vi "Ans_Step2.vi"   [LabVIEW 2012]
uses:
  <vilib>/NXT/Subs/MotorOutput.ctl
types:
  T1 = typedef "MotorOutput.ctl" = u8
  T2 = typedef "LVHSConnector.ctl" = refnum<class "BrickReference.lvclass">
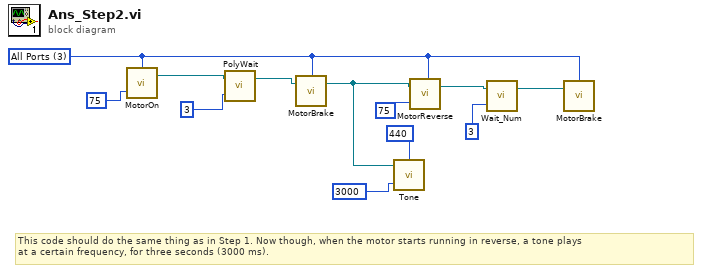
[diagram p0: block diagram]
diagram:
  w3 = T1 3 items=["Port A"=0, "Port B"=1, "Port C"=2, "Ports A & B"=4, "Ports A & C"=5, "Ports B & C"=6, "All Ports"=3] ("Output Port (All Ports)")
  # "This code should do the same thing as in Step 1. Now though, when the motor starts running in reverse, a tone plays\nat a certain frequency, for three seconds (3000 ms)."
  n1 = call <vilib>:"MotorOn.vi"("Power (75)"=75, "Output Port (All Ports)"=w3) -> ("NXT/EV3"=w12:T2)  [unwired: 2 in]
  n2 = call-poly <vilib>:"PolyWait.vi"("Time (1 sec)"=3, "NXT/EV3"=w12) -> ("NXT/EV3"=w10:T2)  [unwired: 2 in]
  n3 = call <vilib>:"MotorBrake.vi"("NXT/EV3"=w10, "Port (All Ports)"=w3) -> ("NXT/EV3"=w9:T2)  [unwired: 2 in]
  n4 = call <vilib>:"Tone.vi"("Duration (500 ms)"=3000, "NXT/EV3"=w9, "Tone (440 Hz)"=440) -> ()  [unwired: 1 in, 1 out]
  n5 = call <vilib>:"MotorReverse.vi"("Power (75)"=75, "NXT/EV3"=w9, "Output Port (All Ports)"=w3) -> ("NXT/EV3"=w5:T2)  [unwired: 1 in]
  n6 = call <vilib>:"Wait_Num.vi"("Time (1 sec)"=3, "NXT/EV3"=w5) -> ("NXT/EV3"=w4:T2)  [unwired: 2 in]
  n7 = call <vilib>:"MotorBrake.vi"("NXT/EV3"=w4, "Port (All Ports)"=w3) -> ()  [unwired: 2 in, 1 out]
